vi "Get Variant.vi"(8 "error in (no error)":errorcluster, 11 "int32 in":refnum<class "string.lvclass">) -> (0 "error out":errorcluster, 2 "Variant":variant, 3 "int32 out":refnum<class "string.lvclass">)   [LabVIEW 2020, in "Protobuf RAW.lvlib" / "string.lvclass"]
uses:
  string.lvclass
  string.lvclass/string.ctl
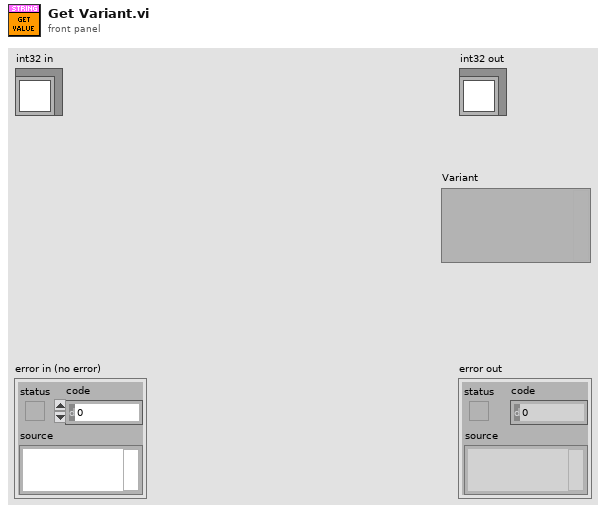
[diagram p1: front panel]
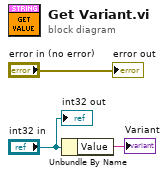
[diagram p0: block diagram]
diagram:
  n1 = Unbundle By Name("int32 in") -> ("Value"=→"Variant":string)
  "error out" <- "error in (no error)"
  "int32 out" <- "int32 in"
